vi "Update NumLevels.vi"(7 "NumLevels":string="2", 8 "error in":errorcluster, 11 "Refnum in":refnum<k20>) -> (0 "error out":errorcluster, 3 "Refnum out":refnum<k20>)   [LabVIEW 2018, in "Serializer.lvclass"]
uses:
  Serializer.lvclass
  <vilib>/xml/Close Reference(Node).vi
  <vilib>/xml/NI_XML.lvlib
  <resource>/objmgr/DOMUserDefRef.rc
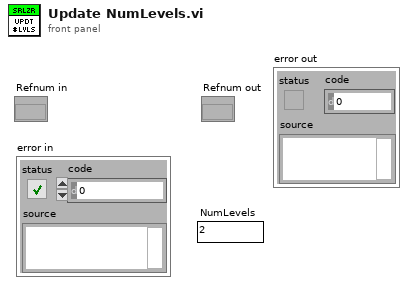
[diagram p1: front panel]
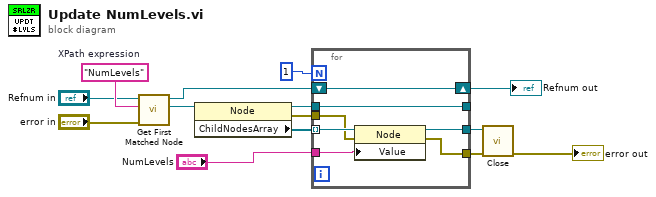
[diagram p0: block diagram]
diagram:
  w14 = "NumLevels"  # XPath expression
  n1 = call <vilib>:"Get First Matched Node.vi"("error in (no error)"="error in", "XPath expression"=w14, "node in"="Refnum in") -> ("node result"=w8:refnum<k20>, "node out"=w11:refnum<k20>)  [unwired: 6 in, 1 out]
  n2 = property class="Node"(reference=w8) -> (reference out=w10:refnum<k20>, error out=w3:errorcluster, "ChildNodesArray"=w6:refnum<k20>[])  [unwired: 1 in]
  n3 = for {
    N: 1 -> [_]
    tunnel: w6 -> [w21] mode=indexing
    tunnel: "NumLevels" -> [w20]
    tunnel: w10 -> [w19]
    tunnel: [w19] -> _
    shift-right: [w18] -> w13
    shift-left: w11 -> [w18]
    tunnel: [w17] -> w4
    tunnel: w3 -> [w16]
    tunnel: [w15] -> w2
    n4 = property class="Node"(reference=w21, error in=w16, "Value"=w20) -> (reference out=w17:refnum<k20>, error out=w15:errorcluster)
  }
  "Refnum out" <- w13
  n5 = call-poly <vilib>:"Close.vi"("error in (no error)"=w2, "node"=w4) -> ("error out"=→"error out":errorcluster)  [unwired: 7 in]
